vi "cDAQ Motor Controller.vi"() -> ()   [LabVIEW 2016]
uses:
  <vilib>/Utility/error.llb/DialogType.ctl
  <vilib>/DAQmx/create/channels.llb/DAQmx Create Channel (DO-Digital Output).vi
  <vilib>/DAQmx/write.llb/DAQmx Write (Digital U8 1Chan 1Samp).vi
panel:
  out "Samples per Channel":u32
  in  "error in":errorcluster
  in  "Slide":u8(slide)=128 scale=0.0..255.0
  in  "Stop":bool
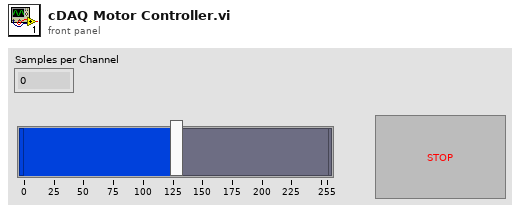
[diagram p1: front panel]
types:
  T1 = typedef "DialogType.ctl" = u16
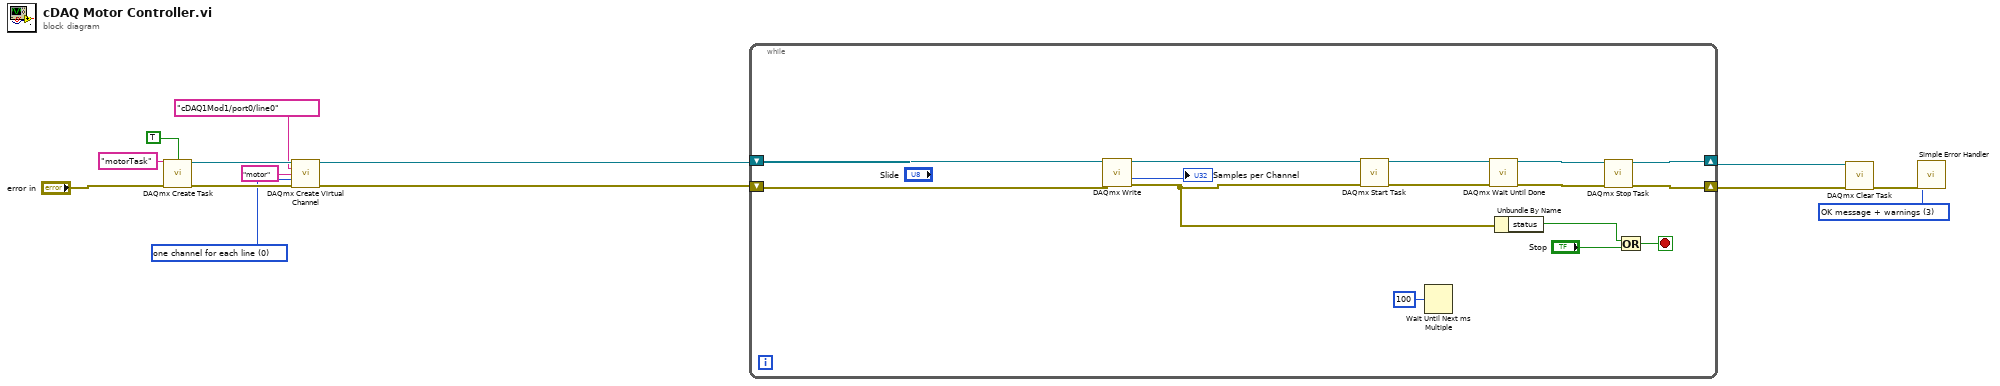
[diagram p0: block diagram]
diagram:
  w5 = 0 items=["one channel for each line", "one channel for all lines"] ("line grouping")
  w13 = T1 3 items=["no dialog", "OK message", "continue or stop message", "OK message + warnings", "continue/stop + warnings"] ("type of dialog (OK msg:1)")
  n1 = call <vilib>:"DAQmx Create Task.vi"("new task name"="motorTask", "auto cleanup"=TRUE, "error in"="error in") -> ("task out"=w12:refnum<k21>, "error out"=w11:errorcluster)  [unwired: 11 in]
  n2 = call-poly <vilib>:"DAQmx Create Virtual Channel.vi"("task in"=w12, "lines"=tag "cDAQ1Mod1/port0/line0", "name to assign"="motor" ("new task name"), "line grouping"=w5, "error in"=w11) -> ("task out"=w4:refnum<k21>, "error out"=w3:errorcluster)  [unwired: 9 in]
  n3 = while {
    shift-right: [w16] -> w2
    shift-left: w4 -> [w24]
    shift-right: [w15] -> w1
    shift-left: w3 -> [w23]
    stop <- w27 stop-if-true
    n4 = call-poly <vilib>:"DAQmx Write.vi"("task/channels in"=w24, "error in"=w23) -> ("task out"=w22:refnum<k21>, "number of samples written per channel"=→"Samples per Channel":u32, "error out"=w21:errorcluster)  [unwired: 11 in]
    n5 = call <vilib>:"DAQmx Start Task.vi"("task/channels in"=w22, "error in"=w21) -> ("task out"=w20:refnum<k21>, "error out"=w19:errorcluster)  [unwired: 12 in]
    n6 = Wait Until Next ms Multiple(millisecond multiple=u32 100) -> ()  [unwired: 1 out]
    n7 = call <vilib>:"DAQmx Wait Until Done.vi"("task/channels in"=w20, "error in"=w19) -> ("task out"=w18:refnum<k21>, "error out"=w17:errorcluster)  [unwired: 12 in]
    n8 = Unbundle By Name(w21) -> ("status"=w29:bool)
    n9 = call <vilib>:"DAQmx Stop Task.vi"("task/channels in"=w18, "error in"=w17) -> ("task out"=w16:refnum<k21>, "error out"=w15:errorcluster)  [unwired: 12 in]
    n10 = Or(x=w29, y="Stop") -> (x .or. y?=w27:bool)
  }
  n11 = call <vilib>:"DAQmx Clear Task.vi"("task in"=w2, "error in"=w1) -> ("error out"=w14:errorcluster)  [unwired: 13 in]
  n12 = call <vilib>:"Simple Error Handler.vi"("type of dialog (OK msg:1)"=w13, "error in (no error)"=w14) -> ()  [unwired: 3 in, 5 out]
